vi "multiple_loops.vi"() -> ()   [LabVIEW 2019]
panel:
  out "result":i32=10000
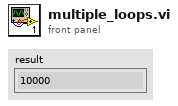
[diagram p1: front panel]
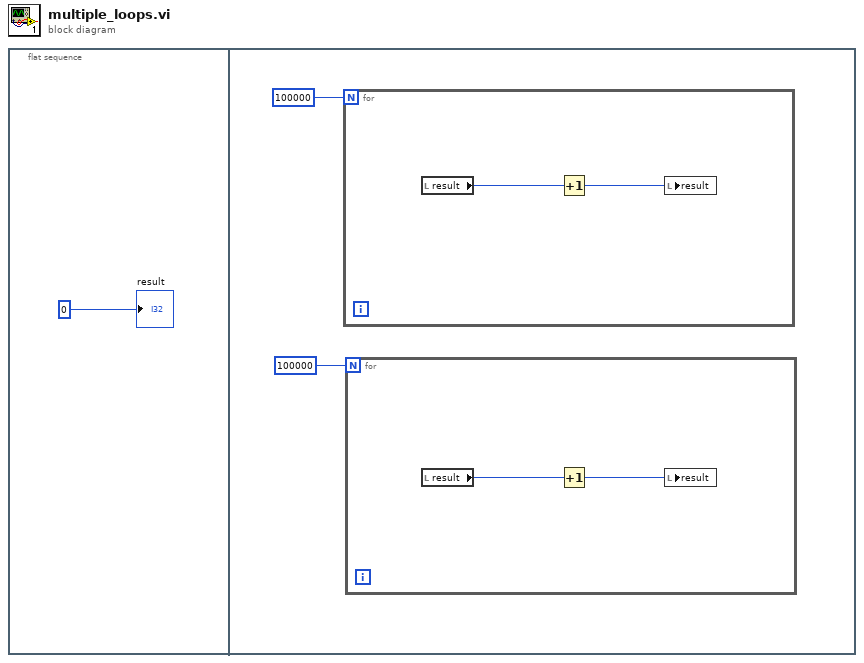
[diagram p0: block diagram]
diagram:
  n1 = flat-sequence {
    frame #0 {
      "result" <- 0 ("result")
    }
    frame #1 {
      n2 = for {
        N: 100000 -> [_]
        n3 = local read "result"() -> (w6:i32)
        n4 = Increment(x=w6) -> (x+1=w7:i32)
        n5 = local write "result"(w7) -> ()
      }
      n6 = for {
        N: 100000 -> [_]
        n7 = local read "result"() -> (w5:i32)
        n8 = Increment(x=w5) -> (x+1=w4:i32)
        n9 = local write "result"(w4) -> ()
      }
    }
  }
